vi "ReversedEngineering CreateTypeDefEdges.vi"(1 "NodeRef":refnum<class "AbstractNode.lvclass">, 2 "AllNodes":refnum<class "AbstractNode.lvclass">[](array[class]), 3 "NodeClassInfo":T1, 4 "TypeDefs":T7[](array[typedef]), 5 "error in (no error)":errorcluster) -> (15 "EdgesCreated":refnum<class "AbstractEdge.lvclass">[](array[class]), 19 "error out":errorcluster)   [LabVIEW 2014]
uses:
  <resource>/Framework/Providers/Open_GDS/UML/AbstractEdge_class/AbstractEdge.lvclass
  <resource>/Framework/Providers/Open_GDS/UML/AbstractNode_class/AbstractNode.lvclass
  <resource>/Framework/Providers/Open_GDS/UML/ReversedEngineering/ReversedEngineering TypeDefType.ctl
  <resource>/Framework/Providers/Open_GDS/UML/ReversedEngineering/ReversedEngineering AttributeInfoType.ctl
  <resource>/Framework/Providers/Open_GDS/ClassProviders/Common/CommonVIs/CommonVIs_AttributeDataType.ctl
  <resource>/Framework/Providers/Open_GDS/UML/UMLEditor/UMLEditor_VisibilityType.ctl
  <resource>/Framework/Providers/Open_GDS/UML/ReversedEngineering/ReversedEngineering ClassInfoType.ctl
  <resource>/Framework/Providers/Open_GDS/UML/ReversedEngineering/ReversedEngineering_ClassDependencyDetailsType.ctl
  <resource>/Framework/Providers/Open_GDS/ClassProviders/Common/ScriptingFunctions/SubVIs/Scripting_ViDependencyType.ctl
  <resource>/Framework/Providers/Open_GDS/UML/ClassNode_class/ExternalSetTypes.ctl
  <resource>/Framework/Providers/Open_GDS/UML/ClassNode_class/ClassNode.lvclass
  <resource>/Framework/Providers/Open_GDS/UML/ClassRelationshipEdge_class/ExternaSetParamType.ctl
  <resource>/Framework/Providers/Open_GDS/UML/ArrowHead_class/ArrowHeadType.ctl
  <resource>/Framework/Providers/Open_GDS/UML/BentStyle_class/BentStyleType.ctl
  <resource>/Framework/Providers/Open_GDS/UML/ReversedEngineering/ReversedEngineering_ViDependencyDetailsType.ctl
  <resource>/Framework/Providers/Open_GDS/UML/ClassRelationshipEdge_class/ClassRelationshipEdge.lvclass
  <resource>/Framework/Providers/Open_GDS/UML/ArrowHead_class/ArrowHead.lvclass
  <resource>/Framework/Providers/Open_GDS/UML/BentStyle_class/BentStyle.lvclass
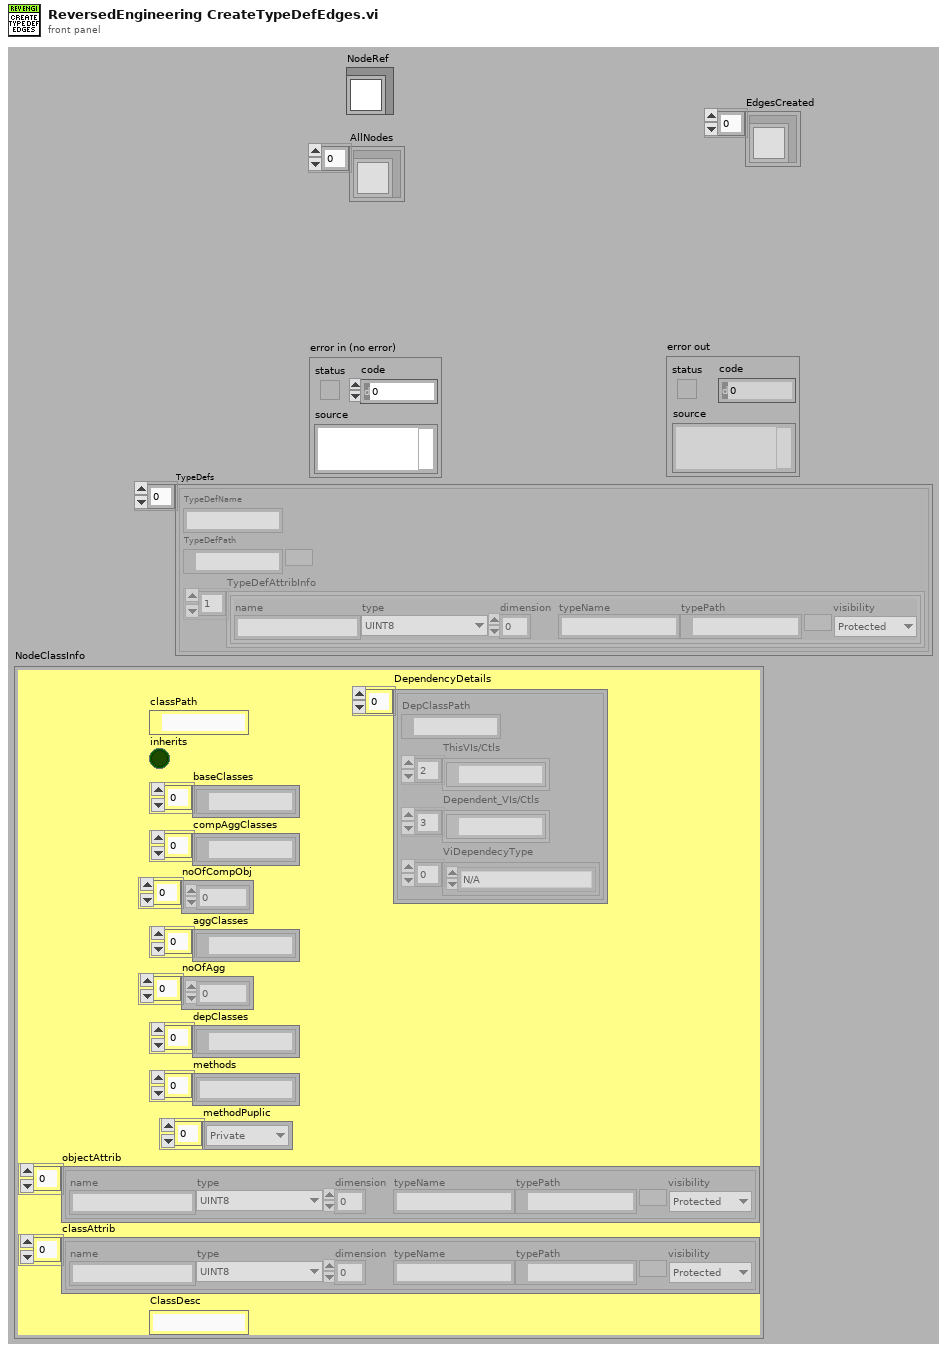
[diagram p1: front panel]
types:
  T1 = typedef "ReversedEngineering ClassInfoType.ctl" = cluster{"classPath":path, "inherits":bool, "baseClasses":path[], "compAggClasses":path[], "noOfCompObj":i32[], "aggClasses":path[], "noOfAgg":i32[], "depClasses":path[], "methods":string[], "methodPuplic":T2[], "objectAttrib":T3[], "classAttrib":T3[], "ClassDesc":string, "DependencyDetails":T5[]}
  T2 = typedef "UMLEditor_VisibilityType.ctl" = enum16{"Public", "Private", "Protected"}
  T3 = typedef "ReversedEngineering AttributeInfoType.ctl" = cluster{"name":string, "type":T4, "dimension":i32, "typeName":string, "typePath":path, "visibility":T2}
  T4 = typedef "CommonVIs_AttributeDataType.ctl" = enum16{"UINT8", "INT8", "UINT16", "INT16", "UINT32", "INT32", "UINT64", "INT64", "SGL", "DBL", "EXT", "CSG", "CDB", "CXT", "TimeStamp", "STRING", "PATH", "BOOL", "ENUM", "RefNum", "VIRefNum", "LabVIEW Class", "Cluster", "Variant", "TypeDef", "Waveform", "LabVIEW Object", "Other", "void"}
  T5 = typedef "ReversedEngineering_ClassDependencyDetailsType.ctl" = cluster{"DepClassPath":path, "ThisVIs/Ctls":path[], "Dependent_VIs/Ctls":path[], "ViDependecyType":T6[]}
  T6 = typedef "Scripting_ViDependencyType.ctl" = enum16{"N/A", "Launches"}
  T7 = typedef "ReversedEngineering TypeDefType.ctl" = cluster{"TypeDefName":string, "TypeDefPath":path, "TypeDefAttribInfo":T3[]}
  T8 = typedef "BentStyle.lvclass/BentStyleType.ctl" = enum16{"STRAIGHT", "HV", "VH", "HVH", "VHV", "ARC"}
  T9 = typedef "ClassRelationshipEdge.lvclass/ExternaSetParamType.ctl" = enum16{"StartLabel", "MidLabel", "EndLabel", "StartNode", "EndNode", "BendType", "StartArrow", "EndArrow"}
  T10 = typedef "ArrowHead.lvclass/ArrowHeadType.ctl" = enum16{"NONE", "TRIANGLE", "BLACK_TRIANGLE", "V", "HALF_V", "DIAMOND", "BLACK_DIAMOND"}
  T11 = typedef "ReversedEngineering_ViDependencyDetailsType.ctl" = cluster{"ThisVIs/Ctls":path[], "Dependent_VIs/Ctls":path[]}
  T12 = typedef "ClassNode.lvclass/ExternalSetTypes.ctl" = enum16{"Name", "Attributes", "Methods", "Position", "ShowMethods", "ShowAttributes", "ClassPath"}
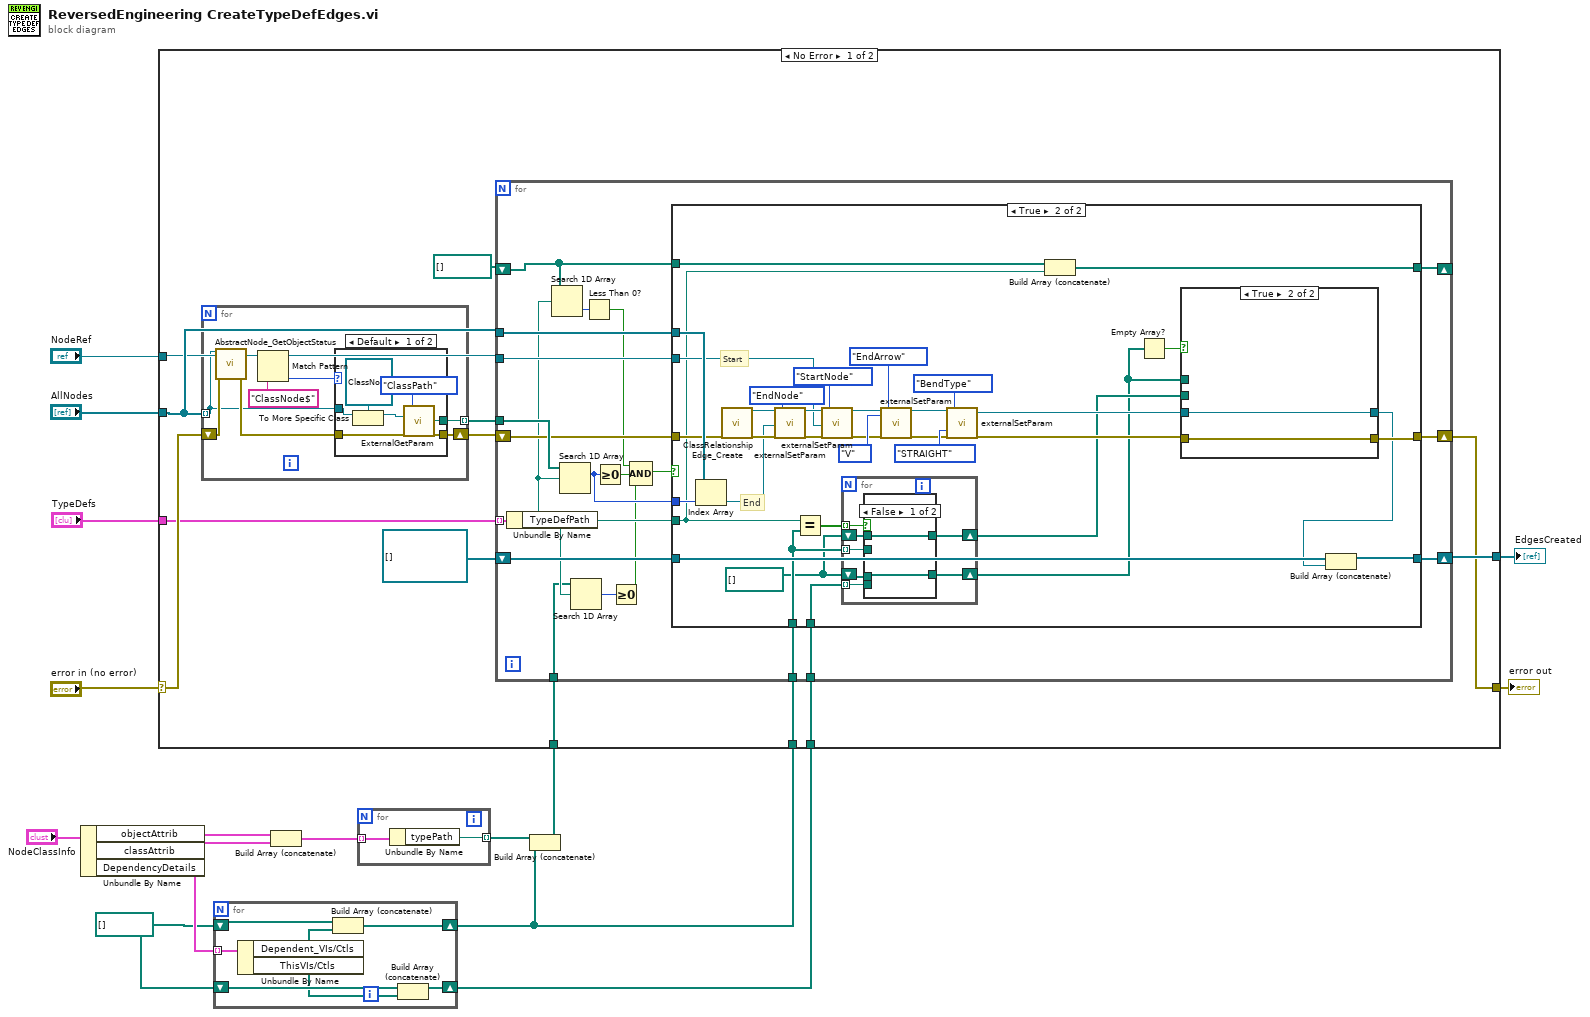
[diagram p0: block diagram]
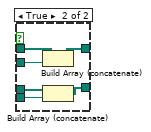
[diagram p3: hidden frame]
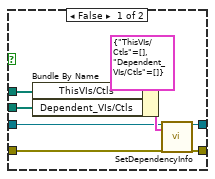
[diagram p4: hidden frame]
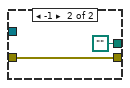
[diagram p5: hidden frame]
diagram:
  w3 = path[] []
  n1 = Unbundle By Name("NodeClassInfo") -> ("objectAttrib"=w9:T3[], "classAttrib"=w8:T3[], "DependencyDetails"=w4:T5[])
  n2 = for {
    tunnel: w4 -> [w23] mode=indexing
    shift-right: [w20] -> w2
    shift-left: w3 -> [w22]
    shift-right: [w18] -> w1
    shift-left: w3 -> [w19]
    n3 = Unbundle By Name(w23) -> ("Dependent_VIs/Ctls"=w21:path[], "ThisVIs/Ctls"=w17:path[])
    n4 = Build Array (concatenate)(w22, w21) -> (w20:path[])
    n5 = Build Array (concatenate)(w19, w17) -> (w18:path[])
  }
  n6 = Build Array (concatenate)(w9, w8) -> (w7:T3[])
  n7 = for {
    tunnel: w7 -> [w25] mode=indexing
    tunnel: [w24] -> w6 mode=indexing
    n8 = Unbundle By Name(w25) -> ("typePath"=w24:path)
  }
  n9 = Build Array (concatenate)(w6, w2) -> (w5:path[])
  n10 = case shown="No Error" "error in (no error)" {
    selector: "error in (no error)" -> [w38 w140]
    tunnel: [w30 w140] -> w15
    tunnel: [w31 _] -> w14
    tunnel: "AllNodes" -> [w34 _]
    tunnel: "NodeRef" -> [w32 _]
    tunnel: "TypeDefs" -> [w37 _]
    tunnel: w5 -> [w28 _]
    tunnel: w2 -> [w27 _]
    tunnel: w1 -> [w26 _]
    frame No Error {
      n11 = for {
        tunnel: w34 -> [w123] mode=indexing
        shift-right: [w129] -> w33
        shift-left: w38 -> [w126]
        tunnel: [w130] -> w36 mode=indexing
        n12 = call <resource>:"AbstractNode_GetObjectStatus.vi"("reference in"=w123, "error in (no error)"=w126) -> ("Class name"=w128:string, "error out"=w125:errorcluster)  [unwired: 16 out]
        n13 = Match Pattern(string=w128, regular expression="ClassNode$") -> (offset past match=w124:i32)  [unwired: 4 out]
        n14 = case shown="Default" w124 {
          tunnel: w123 -> [w132 _]
          tunnel: [w136 path ""] -> w130
          tunnel: [w135 w139] -> w129
          tunnel: w125 -> [w134 w139]
          frame Default {
            n15 = To More Specific Class(target class=refnum<class "ClassNode.lvclass"> refnum ("reference"), reference=w132) -> (specific class reference=w131:refnum<class "ClassNode.lvclass">)  [unwired: 1 in, 1 out]
            n16 = call <resource>:"ExternalGetParam.vi"("reference"=w131, "setParameter"=ExternalSetTypes."ClassPath", "error in (no error)"=w134) -> ("Path"=w136:path, "error out"=w135:errorcluster)  [unwired: 15 out]
          }
          frame -1 {
          }
        }
      }
      n17 = for {
        tunnel: w37 -> [w59] mode=indexing
        tunnel: w36 -> [w58]
        shift-right: [w57] -> w31
        shift-left: refnum<class "AbstractEdge.lvclass">[] [] ("EdgesCreated") -> [w56]
        tunnel: w34 -> [w55]
        shift-right: [w53] -> w30
        shift-left: w33 -> [w54]
        tunnel: w32 -> [w52]
        shift-right: [w45] -> _
        shift-left: path[] [] -> [w46]
        tunnel: w28 -> [w43]
        tunnel: w27 -> [w40]
        tunnel: w26 -> [w39]
        n18 = Unbundle By Name(w59) -> ("TypeDefPath"=w44:path)
        n19 = Search 1D Array(1D array=w46, element=w44) -> (index of element=w48:i32)  [unwired: 1 out]
        n20 = Search 1D Array(1D array=w58, element=w44) -> (index of element=w50:i32)  [unwired: 1 out]
        n21 = Search 1D Array(1D array=w43, element=w44) -> (index of element=w42:i32)  [unwired: 1 out]
        n22 = Less Than 0?(x=w48) -> (x < 0?=w47:bool)
        n23 = Greater Or Equal To 0?(x=w50) -> (x >= 0?=w51:bool)
        n24 = Greater Or Equal To 0?(x=w42) -> (x >= 0?=w41:bool)
        n25 = Compound Arithmetic op=AND(w47, w51, w41) -> (w49:bool)
        n26 = case shown="True" w49 {
          tunnel: [w62 w96] -> w57
          tunnel: w56 -> [w62 w97]
          tunnel: w55 -> [_ w95]
          tunnel: w54 -> [w61 w80]
          tunnel: [w61 w73] -> w53
          tunnel: w52 -> [_ w79]
          tunnel: w50 -> [_ w77]
          tunnel: w46 -> [w60 w76]
          tunnel: [w60 w75] -> w45
          tunnel: w44 -> [_ w70]
          tunnel: w40 -> [_ w68]
          tunnel: w39 -> [_ w67]
          frame False {
          }
          frame True {
            w66 = path[] []
            # "End"
            # "Start"
            n27 = Index Array(array=w95, index=w77) -> (element=w78:refnum<class "AbstractNode.lvclass">)
            n28 = call <resource>:"ClassRelationshipEdge_Create.vi"("error in (no error)"=w80) -> ("reference out"=w81:refnum<class "ClassRelationshipEdge.lvclass">, "error out"=w82:errorcluster)  [unwired: 1 in, 16 out]
            n29 = call-dynamic "externalSetParam.vi"("reference"=w81, "node"=w78, "error in (no error)"=w82, "setParam"=ExternaSetParamType."EndNode") -> ("reference out"=w84:refnum<class "ClassRelationshipEdge.lvclass">, "error out"=w85:errorcluster)  [unwired: 14 in]
            n30 = Equal?(x=w70, y=w68) -> (x = y?=w69:bool[])
            n31 = call-dynamic "externalSetParam.vi"("reference"=w84, "node"=w79, "error in (no error)"=w85, "setParam"=ExternaSetParamType."StartNode") -> ("reference out"=w86:refnum<class "ClassRelationshipEdge.lvclass">, "error out"=w87:errorcluster)  [unwired: 14 in]
            n32 = for {
              shift-right: [w101] -> w65
              shift-left: w66 -> [w102]
              shift-right: [w99] -> w64
              shift-left: w66 -> [w100]
              tunnel: w69 -> [w104] mode=indexing
              tunnel: w68 -> [w103] mode=indexing
              tunnel: w67 -> [w98] mode=indexing
              n33 = case shown="False" w104 {
                tunnel: w103 -> [_ w110]
                tunnel: w102 -> [w106 w112]
                tunnel: [w106 w111] -> w101
                tunnel: w100 -> [w105 w109]
                tunnel: [w105 w108] -> w99
                tunnel: w98 -> [_ w107]
                frame False {
                }
                frame True {
                  n34 = Build Array (concatenate)(w112, w110) -> (w111:path[])
                  n35 = Build Array (concatenate)(w109, w107) -> (w108:path[])
                }
              }
            }
            n36 = call-dynamic "externalSetParam.vi"("reference"=w86, "arrowHead"=ArrowHeadType."V", "error in (no error)"=w87, "setParam"=ExternaSetParamType."EndArrow") -> ("reference out"=w88:refnum<class "ClassRelationshipEdge.lvclass">, "error out"=w89:errorcluster)  [unwired: 14 in]
            n37 = call-dynamic "externalSetParam.vi"("reference"=w88, "bentStyle"=BentStyleType."STRAIGHT", "error in (no error)"=w89, "setParam"=ExternaSetParamType."BendType") -> ("reference out"=w72:refnum<class "ClassRelationshipEdge.lvclass">, "error out"=w74:errorcluster)  [unwired: 14 in]
            n38 = Build Array (concatenate)(w76, w70) -> (w75:path[])
            n39 = Empty Array?(array=w64) -> (empty?=w63:bool)
            n40 = case shown="True" w63 {
              tunnel: [w120 w122] -> w71
              tunnel: [w119 w121] -> w73
              tunnel: w72 -> [w116 w122]
              tunnel: w74 -> [w115 w121]
              tunnel: w65 -> [w114 _]
              tunnel: w64 -> [w113 _]
              frame False {
                n41 = Bundle By Name(cluster=T11 {"ThisVIs/Ctls"=[], "Dependent_VIs/Ctls"=[]} ("DepClass"), "ThisVIs/Ctls"=w113, "Dependent_VIs/Ctls"=w114) -> (w117:T11)
                n42 = call <resource>:"SetDependencyInfo.vi"("reference"=w116, "DepClass"=w117, "error in (no error)"=w115) -> ("reference out"=w120:refnum<class "ClassRelationshipEdge.lvclass">, "error out"=w119:errorcluster)  [unwired: 15 out]
              }
              frame True {
              }
            }
            n43 = Build Array (concatenate)(w97, w71) -> (w96:refnum<class "AbstractEdge.lvclass">[])
          }
        }
      }
    }
    frame Error {
    }
  }
  "error out" <- w15
  "EdgesCreated" <- w14
